vi "ResearcgStandingFrame-V2.2.vi"() -> ()   [LabVIEW 2012]
doc: "Use this template to build a simple state machine design pattern. Each state executes code and determines which state to transition to."
uses:
  controls/State.ctl
  <vilib>/DAQmx/read.llb/DAQmx Read (Analog 2D DBL NChan NSamp).vi
  <vilib>/DAQmx/create/channels.llb/DAQmx Create Channel (AI-Voltage-Basic).vi
  <vilib>/DAQmx/configure/timing.llb/DAQmx Timing (Sample Clock).vi
  <vilib>/DAQmx/create/channels.llb/DAQmx Create Channel (CO-Pulse Generation-Frequency).vi
  <vilib>/DAQmx/configure/timing.llb/DAQmx Timing (Implicit).vi
  <vilib>/DAQmx/miscellaneous.llb/DAQmx Fill In Error Info.vi
  <vilib>/Utility/file.llb/Write To Spreadsheet File (DBL).vi
panel:
  out "refnum out":refnum<file>
  in  "Tab Control":T1(tab)
  in  "?":bool
  out "Center Mass Left Force Plate":cluster{dbl[], dbl[]}(graph)={[-7.494780644696312], [-1.1979086821741642]}
  in  "Save":bool
  in  "stop":bool
  out "Newton Force Readings File Path":path=path "C:/Documents and Settings/z00323/My Documents/Standing Frame/test data/StandingFrameTEST39.dat"
  in  "Newtons":bool
  out "R-FP-Z":dbl
  out "R-FP-Y":dbl
  out "R-FP-X":dbl
  out "R-LC-Z":dbl
  out "R-LC-Y":dbl
  out "R-LC-X":dbl
  out "L-LC-Z":dbl
  out "L-LC-Y":dbl
  out "L-LC-X":dbl
  out "L-FP-X":dbl
  out "L-FP-Y":dbl
  out "L-FP-Z":dbl
  out "String":string caption="Display Unit"
  out "Left Force Plate Z":dbl(slide)=0.43558763460600747 scale=0.0..250.0
  out "Right Force Plate Z":dbl(slide)=0.868584773555102 scale=0.0..250.0
  out "Center Mass Right Force Plate":cluster{dbl[], dbl[]}(graph)
  out "Right Load Cell":cluster{dbl[], dbl[]}(graph)={[0.0, -0.0006862149399022939, 0.0, 0.0], [0.0, 0.005798023167495851, 0.0, 0.0]}
  out "Right Load Cell Z":dbl(slide)=-0.000301685706272135 scale=-50.0..250.0
  out "Left Load Cell Z":dbl(slide)=-0.004073381073294343 scale=-50.0..250.0
  out "Left Load Cell":cluster{dbl[], dbl[]}(graph)={[0.0, -0.0004854170425343219, 0.0, 0.0], [0.0, -0.002818533162237429, 0.0, 0.0]}
  out "Amplitude Unit":string
  out "Right Force PLate Z":dbl(graph)
  out "Left Force Plate Z":dbl(graph)
  out "Right Load Cell Z":dbl(graph)
  out "Right Load Cell Y":dbl(graph)
  out "Right Load Cell X":dbl(graph)
  out "Left Load Cell Z":dbl(graph)
  out "Left Load Cell Y":dbl(graph)
  out "Left Load Cell X":dbl(graph)
  out "Amplitude Unit":string
  out "Loading- Clibration File Path":path
  in  "Save Calibration Results":bool
  in  "Load Previous Calibration Results":bool
  out "Saving- Clibration File Path":path
  out "Baseline Out":dbl[](array[numeric])
  out "Voltages":dbl[](array[numeric])
  in  "New Calibration":bool
  # "FP4"
  # "FP3"
  # "Left Load Cell X\n\nLeft Load Cell Y\n\nLeft Load Cell Z\n\nRight Load Cell X\n\nRight Load Cell Y\n\nRight Load Cell Z"
  # "DAQ Board Connections"
  # "Left Force Plate X1\n\nLeft Force Plate X2\n\nLeft Force Plate Y1\n\nLeft Force Plate Y2\n\nLeft Force Plate Z1\n\nLeft Force Plate Z2\n\nLeft Force Plate Z3\n\nLeft Force Plate Z4"
  # "LX\nLY\nLZ\nRX\nRY\nRZ\nLFX12\nLFX34\nLFY14\nLFY23\nLFZ1\nLFZ2\nLFZ3\nLFZ4\nRFX12\nRFX34\nRFY14\nRFY23\nRFZ1\nRFZ2\nRFZ3\nRFZ4"
  # "32\n33\n34\n35\n36\n37\n0\n1\n2\n3\n4\n5\n6\n7\n16\n17\n18\n19\n20\n21\n22\n23"
  # "Right Force Plate X1\n\nRight Force Plate X2\n\nRight Force Plate Y1\n\nRight Force Plate Y2\n\nRight Force Plate Z1\n\nRight Force Plate Z2\n\nRight Force Plate Z3\n\nRight Force Plate Z4"
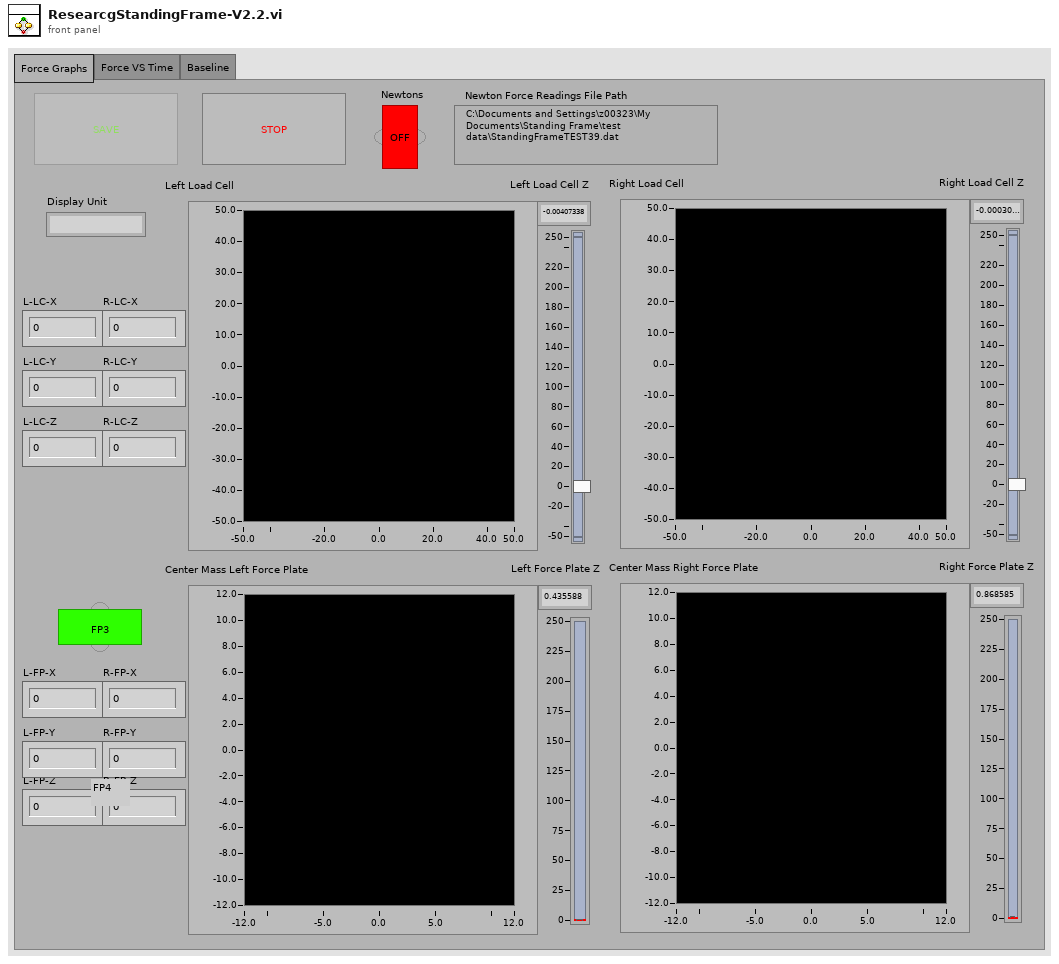
[diagram p1: front panel]
types:
  T1 = enum32{"Force Graphs", "Force VS Time", "Baseline"}
  T2 = typedef "State.ctl" = enum16{"Initialize", "Save", "Main", "Stop"}
  T3 = enum16{"open", "replace", "create", "open or create", "replace or create", "replace or create with confirmation"}
  T4 = enum8{"Enabled", "Disabled", "Disabled and Grayed Out"}
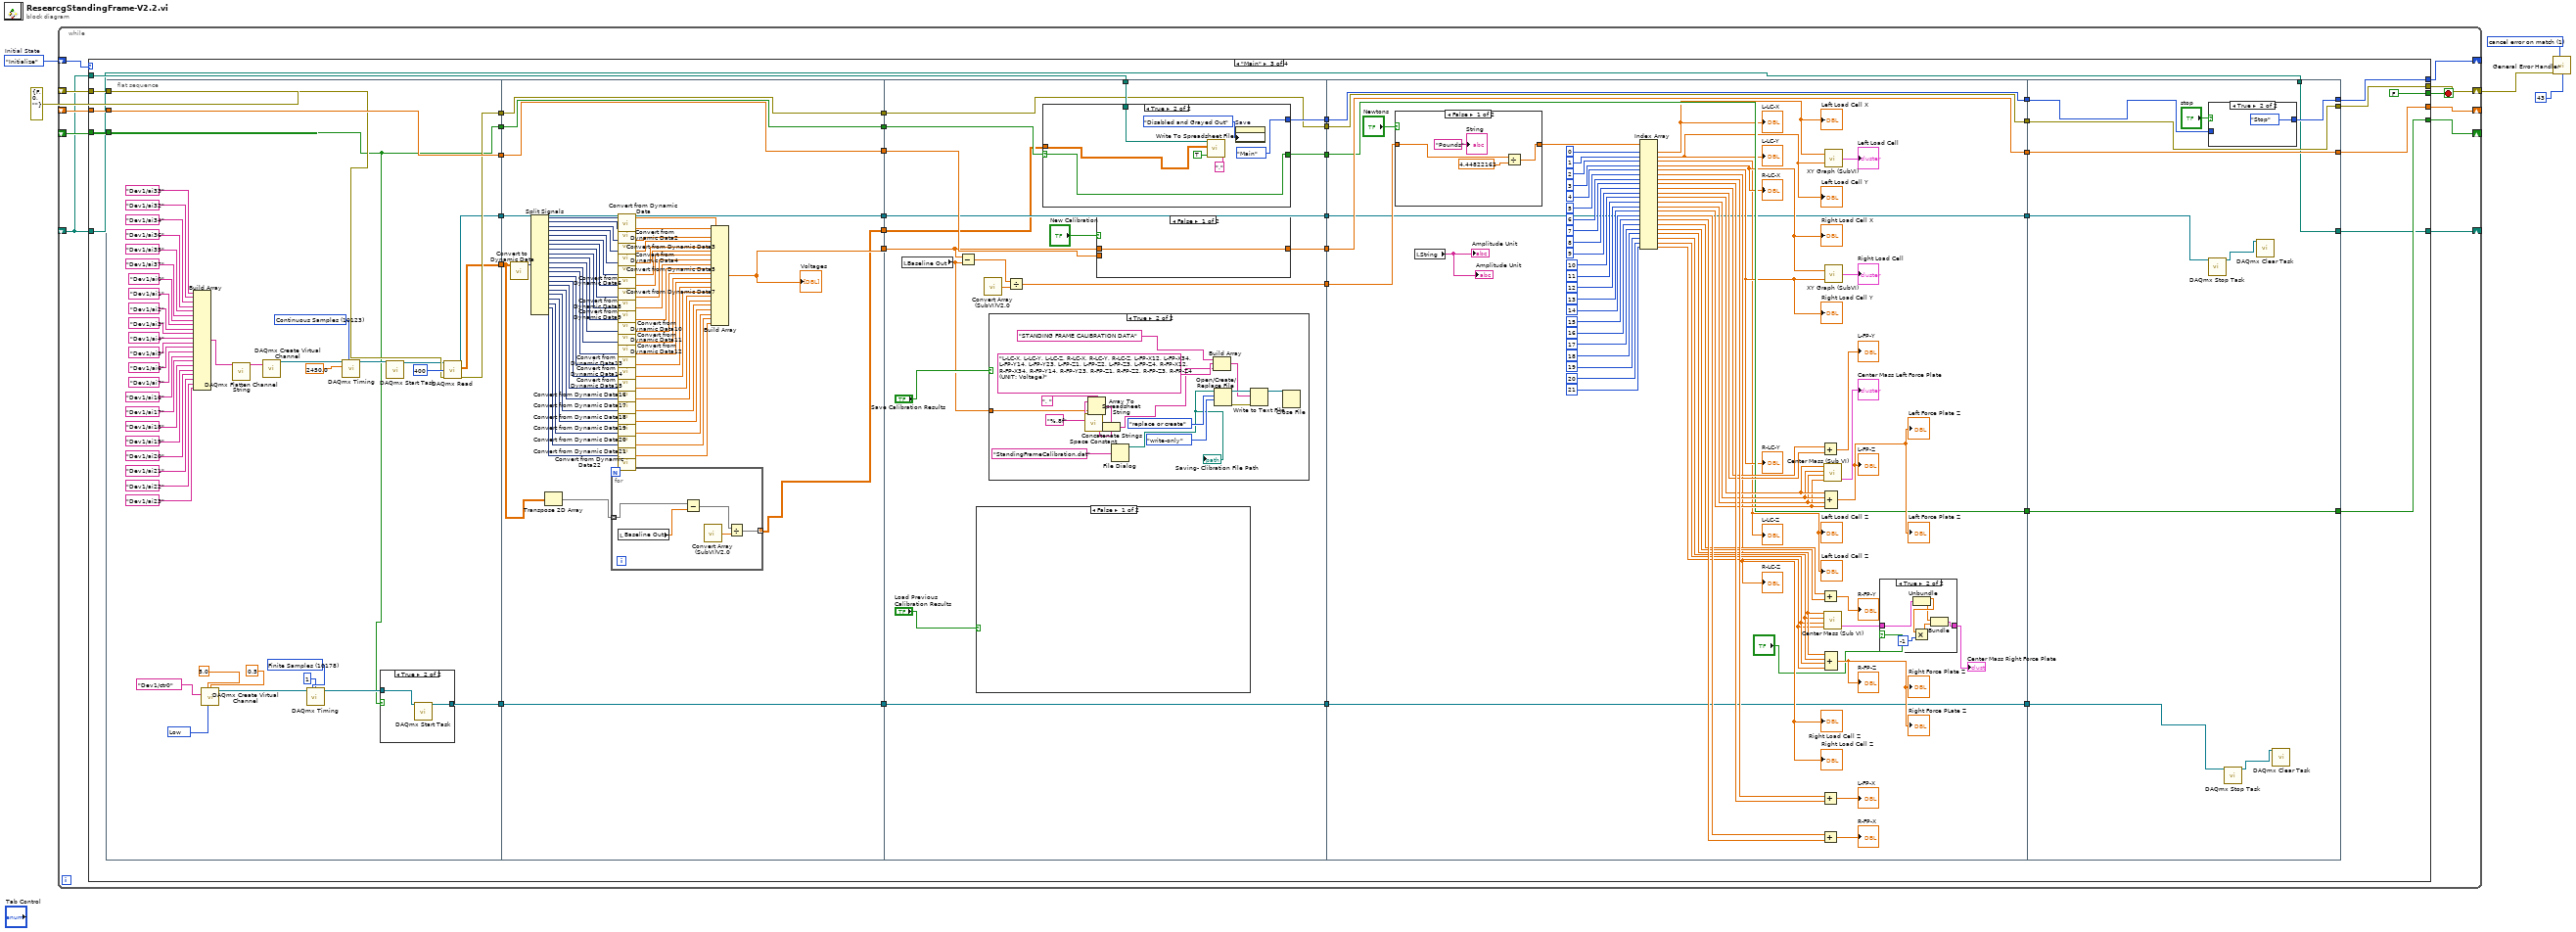
[diagram p0: block diagram]
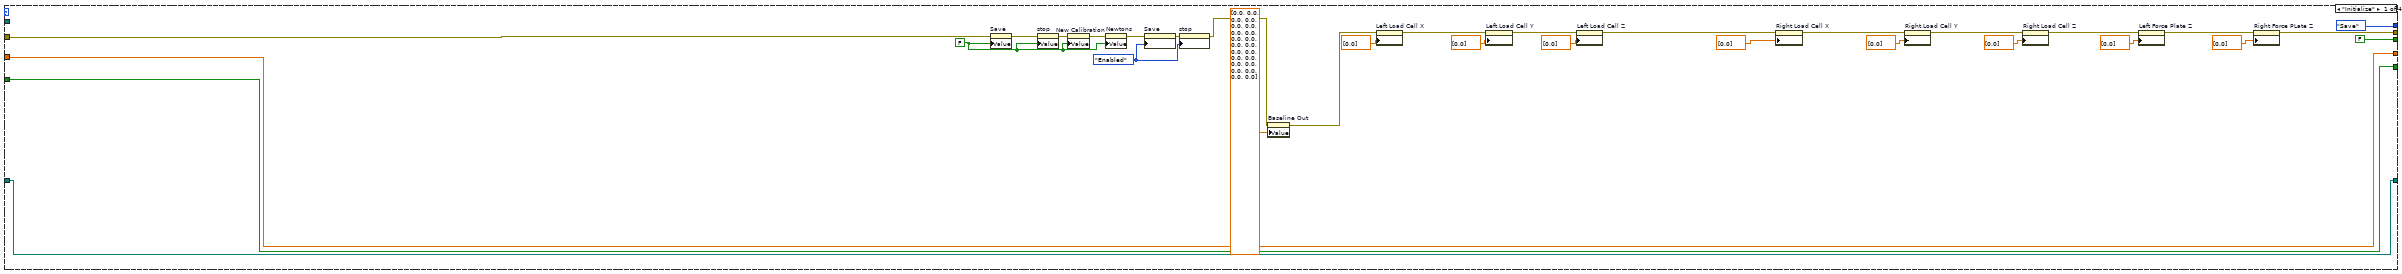
[diagram p2: hidden frame]
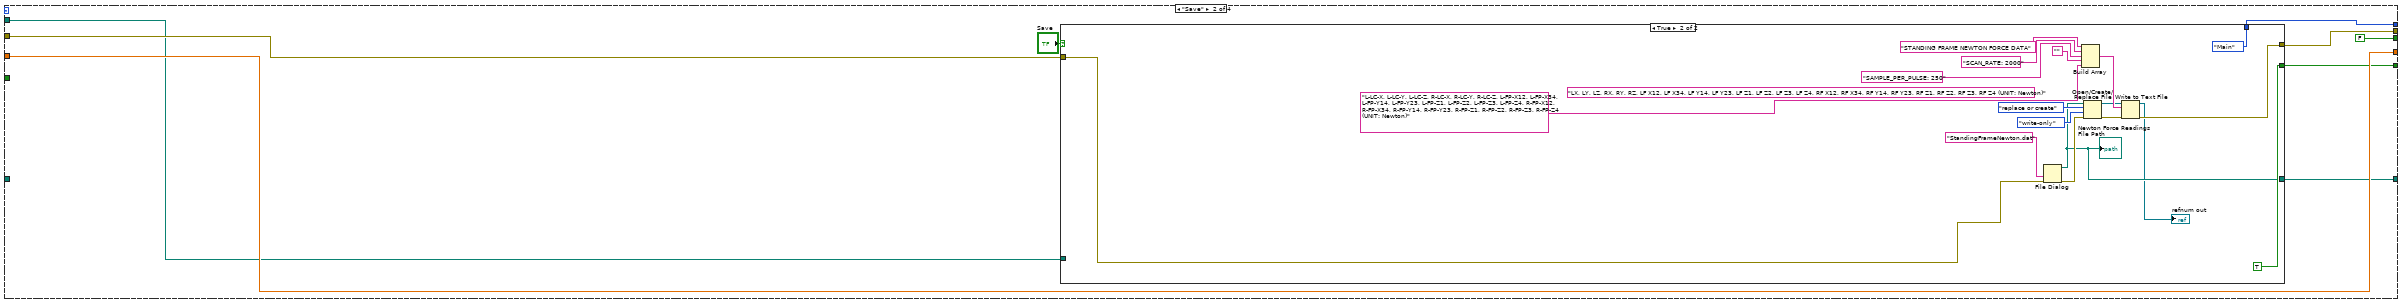
[diagram p3: hidden frame]
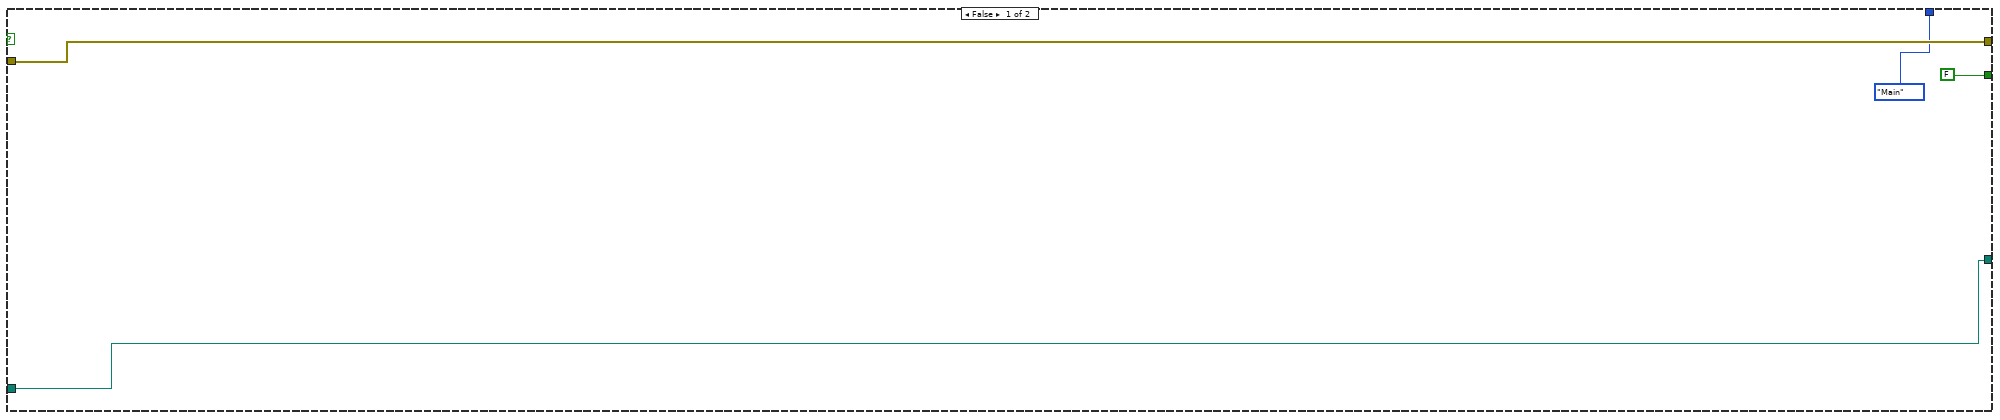
[diagram p4: hidden frame]
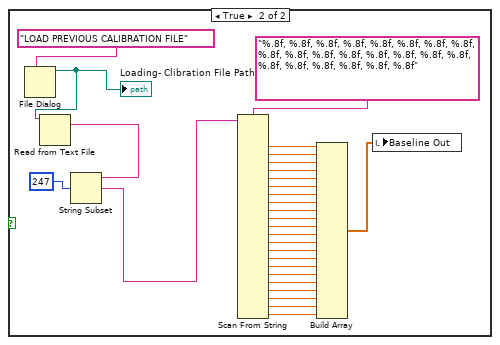
[diagram p6: hidden frame]
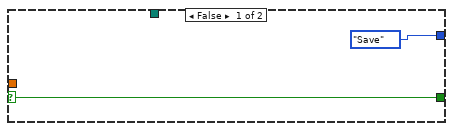
[diagram p8: hidden frame]
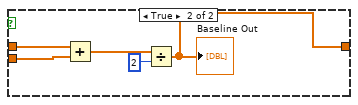
[diagram p9: hidden frame]
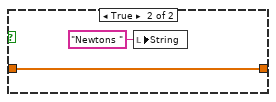
[diagram p11: hidden frame]
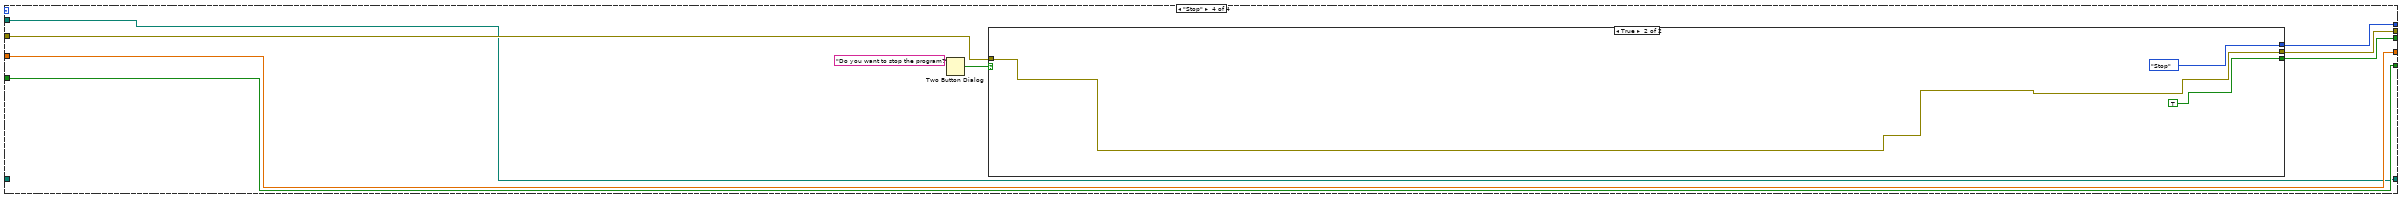
[diagram p13: hidden frame]
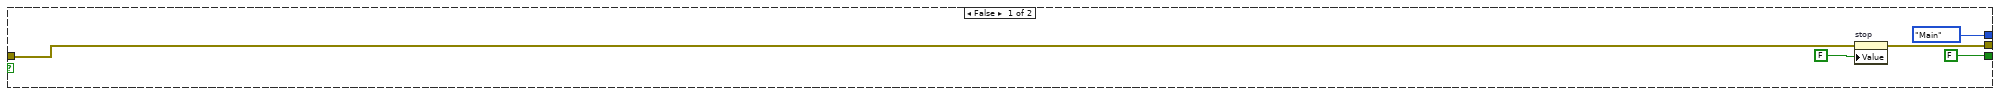
[diagram p14: hidden frame]
diagram:
  w1 = 1 items=["no exception", "cancel error on match", "set error on match"] ("[exception action] (none:0)")
  w5 = State."Initialize"  # Initial State
  n1 = while {
    shift-right: [w16] -> _
    shift-left: w5 -> [w6]
    shift-right: [w13] -> w3
    shift-left: errorcluster {"status"=FALSE, "code"=0, "source"=""} ("error out") -> [w15]
    shift-right: [w11] -> _
    shift-left: _ -> [w12]
    shift-right: [w10] -> _
    shift-left: _ -> [w9]
    shift-right: [w8] -> _
    shift-left: _ -> [w7]
    stop <- w14 stop-if-true
    n2 = case shown="\"Main\"" w6 {
      tunnel: [State."Save" ("Next State") w51 w115 w400] -> w16
      tunnel: [FALSE ("T button?") FALSE FALSE ("T button?") w399] -> w14
      tunnel: w15 -> [w43 w56 w116 w398]
      tunnel: [w20 w55 w107 w397] -> w13
      tunnel: w12 -> [w42 w53 w105 w396]
      tunnel: [w42 w53 w102 w396] -> w11
      tunnel: [w18 w52 w99 w395] -> w10
      tunnel: w9 -> [w18 _ w100 w395]
      tunnel: [w17 w50 w80 w394] -> w8
      tunnel: w7 -> [_ w49 w82 w394]
      tunnel: w7 -> [w17 _ w81 _]
      frame "Initialize" {
        w37 = FALSE ("Begin")
        w46 = T4."Enabled" ("Disabled")
        n3 = property on="Save" class="Bool (strict)"(error in=w43, "Value"=w37) -> (error out=w45:errorcluster)  [unwired: 1 in, 1 out]
        n4 = property on="stop" class="Bool (strict)"(error in=w45, "Value"=w37) -> (error out=w41:errorcluster)  [unwired: 1 in, 1 out]
        n5 = property on="New Calibration" class="Bool (strict)"(error in=w41, "Value"=w37) -> (error out=w39:errorcluster)  [unwired: 1 in, 1 out]
        n6 = property on="Newtons" class="Bool (strict)"(error in=w39, "Value"=w37) -> (error out=w38:errorcluster)  [unwired: 1 in, 1 out]
        n7 = property on="Save" class="Bool (strict)"(error in=w38, "DisabledEnum"=w46) -> (error out=w44:errorcluster)  [unwired: 1 in, 1 out]
        n8 = property on="stop" class="Bool (strict)"(error in=w44, "DisabledEnum"=w46) -> (error out=w19:errorcluster)  [unwired: 1 in, 1 out]
        n9 = property on="Baseline Out" class="Arr (strict)"(error in=w19, "Value"=dbl[] [0.0, 0.0, 0.0, 0.0, 0.0, 0.0, 0.0, 0.0, 0.0, 0.0, 0.0, 0.0, 0.0, 0.0, 0.0, 0.0, 0.0, 0.0, 0.0, 0.0, 0.0, 0.0] ("Baseline Out")) -> (error out=w28:errorcluster)  [unwired: 1 in, 1 out]
        n10 = property on="Left Load Cell X" class="WFChart (strict)"(error in=w28, "History Data"=dbl[] [0.0]) -> (error out=w27:errorcluster)  [unwired: 1 in, 1 out]
        n11 = property on="Left Load Cell Y" class="WFChart (strict)"(error in=w27, "History Data"=dbl[] [0.0]) -> (error out=w26:errorcluster)  [unwired: 1 in, 1 out]
        n12 = property on="Left Load Cell Z" class="WFChart (strict)"(error in=w26, "History Data"=dbl[] [0.0]) -> (error out=w25:errorcluster)  [unwired: 1 in, 1 out]
        n13 = property on="Right Load Cell X" class="WFChart (strict)"(error in=w25, "History Data"=dbl[] [0.0]) -> (error out=w24:errorcluster)  [unwired: 1 in, 1 out]
        n14 = property on="Right Load Cell Y" class="WFChart (strict)"(error in=w24, "History Data"=dbl[] [0.0]) -> (error out=w23:errorcluster)  [unwired: 1 in, 1 out]
        n15 = property on="Right Load Cell Z" class="WFChart (strict)"(error in=w23, "History Data"=dbl[] [0.0]) -> (error out=w22:errorcluster)  [unwired: 1 in, 1 out]
        n16 = property on="Left Force Plate Z" class="WFChart (strict)"(error in=w22, "History Data"=dbl[] [0.0]) -> (error out=w21:errorcluster)  [unwired: 1 in, 1 out]
        n17 = property on="Right Force PLate Z" class="WFChart (strict)"(error in=w21, "History Data"=dbl[] [0.0]) -> (error out=w20:errorcluster)  [unwired: 1 in, 1 out]
      }
      frame "Save" {
        n18 = case shown="True" "Save" {
          tunnel: w56 -> [w61 w62]
          tunnel: [w61 w64] -> w55
          tunnel: [FALSE TRUE] -> w52
          tunnel: [State."Main" ("Next State") State."Main" ("Next State")] -> w51
          tunnel: [w58 w65] -> w50
          tunnel: w49 -> [w58 _]
          frame False {
          }
          frame True {
            (unwired) "LX, LY, LZ, RX, RY, RZ, LF X12, LF X34, LF Y14, LF Y23, LF Z1, LF Z2, LF Z3, LF Z4, RF X12, RF X34, RF Y14, RF Y23, RF Z1, RF Z2, RF Z3, RF Z4 (UNIT: Newton)"
            n19 = File Dialog(8:w62, 9:"StandingFrameNewton.dat" ("default name")) -> (0:w73:errorcluster, 3:w65:path)  [unwired: 2 in, 5 out]
            "Newton Force Readings File Path" <- w65
            n20 = Build Array("STANDING FRAME NEWTON FORCE DATA", "SCAN_RATE: 2000", "SAMPLE_PER_PULSE: 250", "", "L-LC-X, L-LC-Y, L-LC-Z, R-LC-X, R-LC-Y, R-LC-Z, L-FP-X12, L-FP-X34, L-FP-Y14, L-FP-Y23, L-FP-Z1, L-FP-Z2, L-FP-Z3, L-FP-Z4, R-FP-X12, R-FP-X34, R-FP-Y14, R-FP-Y23, R-FP-Z1, R-FP-Z2, R-FP-Z3, R-FP-Z4 (UNIT: Newton)") -> (w76:string[])
            n21 = Open/Create/Replace File(file path (use dialog)=w65, error in=w73, operation (0:open)=T3."replace or create", access (0:read/write)=enum16{"read/write", "read-only", "write-only"}."write-only") -> (refnum out=w75:refnum<file>, error out=w72:errorcluster)  [unwired: 3 out]
            n22 = Write to Text File(file (use dialog)=w75, text=w76, error in=w72) -> (refnum out=→"refnum out":refnum<file>, error out=w64:errorcluster)  [unwired: 1 in, 1 out]
          }
        }
      }
      frame "Main" {
        n23 = flat-sequence {
          tunnel: w116 -> [w147]
          tunnel: [w146] -> w113
          tunnel: [w161] -> w106
          tunnel: w105 -> [w161]
          tunnel: [w120] -> w101
          tunnel: w100 -> [w120]
          tunnel: [w145] -> w89
          tunnel: [w117] -> w88
          tunnel: [w121] -> w84
          tunnel: [w218] -> w96
          tunnel: [w217] -> w95
          tunnel: [w216] -> w94
          tunnel: [w215] -> w93
          tunnel: [w214] -> w90
          tunnel: [w213] -> w85
          tunnel: w84 -> [w213]
          tunnel: w88 -> [w166]
          tunnel: w89 -> [w214]
          tunnel: w101 -> [w215]
          tunnel: w106 -> [w217]
          tunnel: w113 -> [w218]
          tunnel: [w173] -> w83
          tunnel: [w240] -> w112
          tunnel: w96 -> [w224]
          tunnel: [w224] -> w111
          tunnel: [w227] -> w110
          tunnel: w95 -> [w239]
          tunnel: w94 -> [w238]
          tunnel: [w237] -> w104
          tunnel: w93 -> [w234]
          tunnel: [w233] -> w97
          tunnel: [w229] -> w91
          tunnel: w90 -> [w229]
          tunnel: [w228] -> w86
          tunnel: w85 -> [w228]
          tunnel: w83 -> [w226]
          tunnel: w82 -> [w225]
          tunnel: w112 -> [w367]
          tunnel: [w367] -> w109
          tunnel: w111 -> [w316]
          tunnel: w110 -> [w365]
          tunnel: [w316] -> w108
          tunnel: w104 -> [w331]
          tunnel: [w331] -> w103
          tunnel: [w317] -> w98
          tunnel: w97 -> [w317]
          tunnel: [w306] -> w92
          tunnel: w91 -> [w306]
          tunnel: [w305] -> w87
          tunnel: w86 -> [w305]
          tunnel: [w391] -> w115
          tunnel: [w388] -> w107
          tunnel: [w387] -> w102
          tunnel: [w386] -> w99
          tunnel: w81 -> [w381]
          tunnel: [w381] -> w80
          tunnel: w87 -> [w382]
          tunnel: w92 -> [w385]
          tunnel: w98 -> [w386]
          tunnel: w103 -> [w387]
          tunnel: w108 -> [w388]
          tunnel: w109 -> [w389]
          frame #0 {
            w151 = 10178 items=["Finite Samples"=10178, "Continuous Samples"=10123, "Hardware Timed Single Point"=12522] ("sample mode")
            w153 = 10214 items=["High"=10192, "Low"=10214] ("idle state")
            w158 = 10123 items=["Finite Samples"=10178, "Continuous Samples"=10123, "Hardware Timed Single Point"=12522] ("Sample Mode:")
            n24 = Build Array("Dev1/ai33" ("string"), "Dev1/ai32" ("string"), "Dev1/ai34" ("string"), "Dev1/ai36" ("string"), "Dev1/ai35" ("string"), "Dev1/ai37" ("string"), "Dev1/ai0" ("string"), "Dev1/ai1" ("string"), "Dev1/ai2" ("string"), "Dev1/ai3" ("string"), "Dev1/ai4" ("string"), "Dev1/ai5" ("string"), "Dev1/ai6" ("string"), "Dev1/ai7" ("string"), "Dev1/ai16" ("string"), "Dev1/ai17" ("string"), "Dev1/ai18" ("string"), "Dev1/ai19" ("string"), "Dev1/ai20" ("string"), "Dev1/ai21" ("string"), "Dev1/ai22" ("string"), "Dev1/ai23" ("string")) -> (w118:string[])
            n25 = call-poly <vilib>:"DAQmx Create Virtual Channel.vi"("frequency"=5.0, "duty cycle"=0.5, "counter"=tag "Dev1/ctr0" ("Pulse Output Channel"), "idle state"=w153) -> ("task out"=w152:refnum<k21>)  [unwired: 10 in, 1 out]
            n26 = call <vilib>:"DAQmx Flatten Channel String.vi"("names in"=w118) -> ("names out"=w160:string)  [unwired: 13 in, 1 out]
            n27 = call-poly <vilib>:"DAQmx Create Virtual Channel.vi"("physical channels"=w160) -> ("task out"=w159:refnum<k21>)  [unwired: 13 in, 1 out]
            n28 = call-poly <vilib>:"DAQmx Timing.vi"("task/channels in"=w152, "sample mode"=w151, "samples per channel"=1) -> ("task out"=w122:refnum<k21>)  [unwired: 11 in, 1 out]
            n29 = call-poly <vilib>:"DAQmx Timing.vi"("task/channels in"=w159, "sample mode"=w158, "rate"=sgl 2450.0 ("Scan Rate:")) -> ("task out"=w149:refnum<k21>)  [unwired: 11 in, 1 out]
            n30 = case shown="True" w120 {
              tunnel: w122 -> [w162 w164]
              tunnel: [w162 w163] -> w121
              frame False {
              }
              frame True {
                n31 = call <vilib>:"DAQmx Start Task.vi"("task/channels in"=w164) -> ("task out"=w163:refnum<k21>)  [unwired: 13 in, 1 out]
              }
            }
            n32 = call <vilib>:"DAQmx Start Task.vi"("task/channels in"=w149) -> ("task out"=w119:refnum<k21>)  [unwired: 13 in, 1 out]
            n33 = call-poly <vilib>:"DAQmx Read.vi"("task/channels in"=w119, "number of samples per channel"=400, "error in"=w147) -> ("task out"=w145:refnum<k21>, "data"=w117:dbl[][], "error out"=w146:errorcluster)  [unwired: 10 in]
          }
          frame #1 {
            n34 = call "Convert to Dynamic Data"("2D Array"=w166) -> ("Dynamic Data Type"=w174:dynamicdata)  [unwired: 3 in]
            n35 = Split Signals(w174) -> (w212:dynamicdata, w211:dynamicdata, w210:dynamicdata, w209:dynamicdata, w208:dynamicdata, w207:dynamicdata, w206:dynamicdata, w205:dynamicdata, w204:dynamicdata, w203:dynamicdata, w202:dynamicdata, w201:dynamicdata, w200:dynamicdata, w199:dynamicdata, w198:dynamicdata, w197:dynamicdata, w196:dynamicdata, w195:dynamicdata, w194:dynamicdata, w193:dynamicdata, w192:dynamicdata, w191:dynamicdata)  [unwired: 22 in]
            n36 = Transpose 2D Array(2D array=w166) -> (transposed array=w167:dbl[][])
            n37 = for {
              tunnel: w167 -> [w219] mode=indexing
              tunnel: [w220] -> w173 mode=indexing
              n38 = local read "Baseline Out"() -> (w223:dbl[])
              n39 = Subtract(x=w219, y=w223) -> (x-y=w222:dbl[])
              n40 = call "Convert Array  (SubVI)V2.0.vi"() -> ("Conversion Array"=w221:dbl[])  [unwired: 1 in]
              n41 = Divide(x=w222, y=w221) -> (x/y=w220:dbl[])
            }
            n42 = call "Convert from Dynamic Data"("Dynamic Data Type"=w212) -> ("Scalar"=w171:dbl)  [unwired: 3 in]
            n43 = call "Convert from Dynamic Data2"("Dynamic Data Type"=w211) -> ("Scalar"=w172:dbl)  [unwired: 3 in]
            n44 = call "Convert from Dynamic Data3"("Dynamic Data Type"=w210) -> ("Scalar"=w165:dbl)  [unwired: 3 in]
            n45 = call "Convert from Dynamic Data4"("Dynamic Data Type"=w209) -> ("Scalar"=w170:dbl)  [unwired: 3 in]
            n46 = call "Convert from Dynamic Data5"("Dynamic Data Type"=w208) -> ("Scalar"=w169:dbl)  [unwired: 3 in]
            n47 = call "Convert from Dynamic Data6"("Dynamic Data Type"=w207) -> ("Scalar"=w168:dbl)  [unwired: 3 in]
            n48 = call "Convert from Dynamic Data7"("Dynamic Data Type"=w206) -> ("Scalar"=w179:dbl)  [unwired: 3 in]
            n49 = call "Convert from Dynamic Data8"("Dynamic Data Type"=w205) -> ("Scalar"=w180:dbl)  [unwired: 3 in]
            n50 = call "Convert from Dynamic Data9"("Dynamic Data Type"=w204) -> ("Scalar"=w181:dbl)  [unwired: 3 in]
            n51 = call "Convert from Dynamic Data10"("Dynamic Data Type"=w203) -> ("Scalar"=w182:dbl)  [unwired: 3 in]
            n52 = call "Convert from Dynamic Data11"("Dynamic Data Type"=w202) -> ("Scalar"=w178:dbl)  [unwired: 3 in]
            n53 = call "Convert from Dynamic Data12"("Dynamic Data Type"=w201) -> ("Scalar"=w177:dbl)  [unwired: 3 in]
            n54 = call "Convert from Dynamic Data13"("Dynamic Data Type"=w200) -> ("Scalar"=w183:dbl)  [unwired: 3 in]
            n55 = call "Convert from Dynamic Data14"("Dynamic Data Type"=w199) -> ("Scalar"=w176:dbl)  [unwired: 3 in]
            n56 = call "Convert from Dynamic Data15"("Dynamic Data Type"=w198) -> ("Scalar"=w175:dbl)  [unwired: 3 in]
            n57 = call "Convert from Dynamic Data16"("Dynamic Data Type"=w197) -> ("Scalar"=w184:dbl)  [unwired: 3 in]
            n58 = call "Convert from Dynamic Data17"("Dynamic Data Type"=w196) -> ("Scalar"=w185:dbl)  [unwired: 3 in]
            n59 = call "Convert from Dynamic Data18"("Dynamic Data Type"=w195) -> ("Scalar"=w186:dbl)  [unwired: 3 in]
            n60 = call "Convert from Dynamic Data19"("Dynamic Data Type"=w194) -> ("Scalar"=w187:dbl)  [unwired: 3 in]
            n61 = call "Convert from Dynamic Data20"("Dynamic Data Type"=w193) -> ("Scalar"=w188:dbl)  [unwired: 3 in]
            n62 = call "Convert from Dynamic Data21"("Dynamic Data Type"=w192) -> ("Scalar"=w189:dbl)  [unwired: 3 in]
            n63 = call "Convert from Dynamic Data22"("Dynamic Data Type"=w191) -> ("Scalar"=w190:dbl)  [unwired: 3 in]
            n64 = Build Array(w171, w172, w165, w170, w169, w168, w179, w180, w181, w182, w178, w177, w183, w176, w175, w184, w185, w186, w187, w188, w189, w190) -> (w216:dbl[])
            "Voltages" <- w216
          }
          frame #2 {
            n65 = local read "Baseline Out"() -> (w231:dbl[])
            n66 = Subtract(x=w238, y=w231) -> (x-y=w236:dbl[])
            n67 = case shown="False" "Load Previous Calibration Results" {
              frame False {
              }
              frame True {
                n68 = File Dialog(7:"LOAD PREVIOUS CALIBRATION FILE") -> (3:w242:path)  [unwired: 2 in, 7 out]
                "Loading- Clibration File Path" <- w242
                n69 = Read from Text File(file (use dialog)=w242) -> (text=w248:string)  [unwired: 3 in, 3 out]
                n70 = String Subset(string=w248, offset (0)=247) -> (substring=w246:string)  [unwired: 1 in]
                n71 = Scan From String(format string="%.8f, %.8f, %.8f, %.8f, %.8f, %.8f, %.8f, %.8f, %.8f, %.8f, %.8f, %.8f, %.8f, %.8f, %.8f, %.8f, %.8f, %.8f, %.8f, %.8f, %.8f, %.8f", input string=w246) -> (output 1=w270:dbl, output 2=w269:dbl, output 3=w268:dbl, output 4=w267:dbl, output 5=w266:dbl, output 6=w265:dbl, output 7=w264:dbl, output 8=w263:dbl, output 9=w262:dbl, output 10=w261:dbl, output 11=w260:dbl, output 12=w259:dbl, output 13=w258:dbl, output 14=w257:dbl, output 15=w256:dbl, output 16=w255:dbl, output 17=w254:dbl, output 18=w253:dbl, output 19=w252:dbl, output 20=w251:dbl, output 21=w250:dbl, output 22=w249:dbl)  [unwired: 24 in, 3 out]
                n72 = Build Array(w270, w269, w268, w267, w266, w265, w264, w263, w262, w261, w260, w259, w258, w257, w256, w255, w254, w253, w252, w251, w250, w249) -> (w245:dbl[])
                n73 = local write "Baseline Out"(w245) -> ()
              }
            }
            n74 = call "Convert Array  (SubVI)V2.0.vi"() -> ("Conversion Array"=w235:dbl[])  [unwired: 1 in]
            n75 = case shown="True" "Save Calibration Results" {
              tunnel: w231 -> [_ w279]
              frame False {
              }
              frame True {
                n76 = call <vilib>:"Space Constant.vi"() -> ("String"=w274:string)
                n77 = Array To Spreadsheet String(delimiter (Tab)=", ", array=w279, 3:"%.8f") -> (spreadsheet string=w273:string)
                n78 = Concatenate Strings(w274, w273) -> (w272:string)
                n79 = File Dialog(9:"StandingFrameCalibration.dat" ("default name")) -> (3:w271:path)  [unwired: 2 in, 7 out]
                "Saving- Clibration File Path" <- w271
                n80 = Build Array("STANDING FRAME CALIBRATION DATA", "L-LC-X, L-LC-Y, L-LC-Z, R-LC-X, R-LC-Y, R-LC-Z, L-FP-X12, L-FP-X34, L-FP-Y14, L-FP-Y23, L-FP-Z1, L-FP-Z2, L-FP-Z3, L-FP-Z4, R-FP-X12, R-FP-X34, R-FP-Y14, R-FP-Y23, R-FP-Z1, R-FP-Z2, R-FP-Z3, R-FP-Z4 (UNIT: Voltage)", w272) -> (w284:string[])
                n81 = Open/Create/Replace File(file path (use dialog)=w271, operation (0:open)=T3."replace or create", access (0:read/write)=enum16{"read/write", "read-only", "write-only"}."write-only") -> (refnum out=w285:refnum<file>, error out=w286:errorcluster)  [unwired: 1 in, 3 out]
                n82 = Write to Text File(file (use dialog)=w285, text=w284, error in=w286) -> (refnum out=w277:refnum<file>)  [unwired: 1 in, 2 out]
                n83 = Close File(refnum=w277) -> ()  [unwired: 1 in, 2 out]
              }
            }
            n84 = Divide(x=w236, y=w235) -> (x/y=w227:dbl[])
            n85 = case shown="True" w234 {
              selector: w234 -> [w287 w293]
              tunnel: [State."Save" ("(Value Not Used)") State."Main" ("(Value Not Used)")] -> w240
              tunnel: w226 -> [_ w292]
              tunnel: [w287 w293] -> w233
              tunnel: w225 -> [_ w290]
              frame False {
              }
              frame True {
                n86 = call-poly <vilib>:"Write To Spreadsheet File.vi"("delimiter (\\t)"="," ("delimiter (\\t)"), "append to file? (new file:F)"=TRUE, "2D data"=w292, "file path (dialog if empty)"=w290) -> ()  [unwired: 4 in, 1 out]
                n87 = property on="Save" class="Bool (strict)"("DisabledEnum"=T4."Disabled and Grayed Out" ("Disabled")) -> ()  [unwired: 2 in, 2 out]
              }
            }
            n88 = case shown="False" "New Calibration" {
              tunnel: w239 -> [_ w297]
              tunnel: w238 -> [w296 w299]
              tunnel: [w296 w298] -> w237
              frame False {
              }
              frame True {
                n89 = Add(x=w299, y=w297) -> (x+y=w301:dbl[])
                n90 = Divide(x=w301, y=2) -> (x/y=w298:dbl[])
                "Baseline Out" <- w298
              }
            }
          }
          frame #3 {
            n91 = case shown="False" "Newtons" {
              tunnel: w365 -> [w377 w379]
              tunnel: [w376 w379] -> w364
              frame False {
                n92 = Divide(x=w377, y=4.44822162) -> (x/y=w376:dbl[])
                "String" <- "Pounds" ("String")
              }
              frame True {
                n93 = local write "String"("Newtons " ("String")) -> ()
              }
            }
            n94 = local read "String"() -> (→"Amplitude Unit" →"Amplitude Unit":string)
            n95 = Index Array(array=w364, index #1=0 ("index (row)"), index #2=1 ("index (row)"), index #3=2 ("index (row)"), index #4=3 ("index (row)"), index #5=4 ("index (row)"), index #6=5 ("index (row)"), index #7=6 ("index (row)"), index #8=7 ("index (row)"), index #9=8 ("index (row)"), index #10=9 ("index (row)"), index #11=10 ("index (row)"), index #12=11 ("index (row)"), index #13=12 ("index (row)"), index #14=13 ("index (row)"), index #15=14 ("index (row)"), index #16=15 ("index (row)"), index #17=16 ("index (row)"), index #18=17 ("index (row)"), index #19=18 ("index (row)"), index #20=19 ("index (row)"), index #21=20 ("index (row)"), index #22=21 ("index (row)")) -> (element #1=w310:dbl, element #2=w311:dbl, element #3=→"L-LC-Z" →"Left Load Cell Z" →"Left Load Cell Z":dbl, element #4=w312:dbl, element #5=w313:dbl, element #6=→"R-LC-Z" →"Right Load Cell Z" →"Right Load Cell Z":dbl, element #7=w341:dbl, element #8=w340:dbl, element #9=w338:dbl, element #10=w337:dbl, element #11=w327:dbl, element #12=w326:dbl, element #13=w325:dbl, element #14=w324:dbl, element #15=w335:dbl, element #16=w334:dbl, element #17=w333:dbl, element #18=w332:dbl, element #19=w323:dbl, element #20=w322:dbl, element #21=w321:dbl, element #22=w320:dbl)
            "L-LC-X" <- w310
            "L-LC-Y" <- w311
            "R-LC-X" <- w312
            "R-LC-Y" <- w313
            "Left Load Cell X" <- w310
            "Left Load Cell Y" <- w311
            "Right Load Cell X" <- w312
            "Right Load Cell Y" <- w313
            n96 = Add(x=w338, y=w337) -> (x+y=→"L-FP-Y":dbl)
            n97 = Add(x=w333, y=w332) -> (x+y=→"R-FP-Y":dbl)
            n98 = Add(x=w341, y=w340) -> (x+y=→"L-FP-X":dbl)
            n99 = Add(x=w335, y=w334) -> (x+y=→"R-FP-X":dbl)
            n100 = call "Center Mass (Sub VI).vi"("Z4"=w324, "Z3"=w325, "Z2"=w326, "Z1"=w327) -> ("XY Graph"=→"Center Mass Left Force Plate":cluster{dbl[], dbl[]})  [unwired: 2 in]
            n101 = call "Center Mass (Sub VI).vi"("Z4"=w320, "Z3"=w321, "Z2"=w322, "Z1"=w323) -> ("XY Graph"=w302:cluster{dbl[], dbl[]})  [unwired: 2 in]
            n102 = call "XY Graph (SubVI).vi"("Y"=w311, "X"=w310) -> ("XY Graph"=→"Left Load Cell":cluster{"array":dbl[], "array":dbl[]})
            n103 = call "XY Graph (SubVI).vi"("Y"=w313, "X"=w312) -> ("XY Graph"=→"Right Load Cell":cluster{"array":dbl[], "array":dbl[]})
            n104 = Compound Arithmetic op=ADD(w327, w326, w325, w324) -> (→"L-FP-Z" →"Left Force Plate Z" →"Left Force Plate Z":dbl)
            n105 = Compound Arithmetic op=ADD(w323, w322, w321, w320) -> (→"R-FP-Z" →"Right Force PLate Z" →"Right Force Plate Z":dbl)
            n106 = case shown="True" "?" {
              tunnel: [w368 w369] -> w303
              tunnel: w302 -> [w368 w374]
              frame False {
              }
              frame True {
                n107 = Unbundle(w374) -> (w373:dbl[], w372:dbl[])
                n108 = Multiply(x=w373, y=-1) -> (x*y=w371:dbl[])
                n109 = Bundle(w372, w371) -> (w369:cluster{dbl[], dbl[]})  [unwired: 1 in]
              }
            }
            "Center Mass Right Force Plate" <- w303
          }
          frame #4 {
            n110 = call <vilib>:"DAQmx Stop Task.vi"("task/channels in"=w385) -> ("task out"=w384:refnum<k21>)  [unwired: 13 in, 1 out]
            n111 = case shown="True" "stop" {
              tunnel: [w392 State."Stop" ("(Value Not Used)")] -> w391
              tunnel: w389 -> [w392 _]
              frame False {
              }
              frame True {
              }
            }
            n112 = call <vilib>:"DAQmx Stop Task.vi"("task/channels in"=w382) -> ("task out"=w383:refnum<k21>)  [unwired: 13 in, 1 out]
            n113 = call <vilib>:"DAQmx Clear Task.vi"("task in"=w384) -> ()  [unwired: 14 in, 1 out]
            n114 = call <vilib>:"DAQmx Clear Task.vi"("task in"=w383) -> ()  [unwired: 14 in, 1 out]
          }
        }
      }
      frame "Stop" {
        n115 = Two Button Dialog(message="Do you want to stop the program?") -> (T button?=w401:bool)  [unwired: 2 in]
        n116 = case shown="True" w401 {
          tunnel: [FALSE TRUE] -> w399
          tunnel: [State."Main" ("(Value Not Used)") State."Stop" ("(Value Not Used)")] -> w400
          tunnel: w398 -> [w403 w408]
          tunnel: [w404 w408] -> w397
          frame False {
            n117 = property on="stop" class="Bool (strict)"(error in=w403, "Value"=FALSE ("stop")) -> (error out=w404:errorcluster)  [unwired: 1 in, 1 out]
          }
          frame True {
          }
        }
      }
    }
  }
  n118 = call <vilib>:"General Error Handler.vi"("error in (no error)"=w3, "[exception action] (none:0)"=w1, "[exception code]"=43) -> ()  [unwired: 8 in, 5 out]
